vi "ObjDet_Read_Dataset_Single.vi"(6 "Dims(C,H,W)":T1={"C"=-1, "H"=-1, "W"=-1}, 7 "Unique labels":string[](array[string]), 8 "error in (no error)":errorcluster, 9 "Dataset Path (Images)":path=path "D:/DNN/Nuts_Bolts/Orig/1_Test/Images", 11 "Annotations Path":path=path "D:/DNN/Nuts_Bolts/Orig/1_Test/Annotations") -> (0 "error out":errorcluster, 2 "Anchors":dbl[][](array[numeric]), 3 "NN_DataSet(In3D_OutBBox)":T2={"Inputs Ref."=variant(refnum<data-value> refnum), "Dataset_Size"=0, "Dims_In"={"C"=0, "H"=0, "W"=0}, "Outputs Refs"=refnum, "No of Classes "=0, "Labels"=[], "File Paths"=[]})   [LabVIEW 2020]
uses:
  <vilib>/Ngene/Deep Learning Toolkit/Toolkit/NN_Data/API/DataSet/DataSet_Types/NN_DataSet(In3D_OutBBox).ctl
  <vilib>/Ngene/Deep Learning Toolkit/Toolkit/NN_Data/API/NN_Dims(C,H,W).ctl
  <vilib>/Ngene/Deep Learning Toolkit/Toolkit/NN_Data/Controls/DataRef_Types/1D/NN_Data_ref(1D_BBox).ctl
  <vilib>/Ngene/Deep Learning Toolkit/Toolkit/NN_Data/API/Data/Detection_Types/NN_Image_Annotations.ctl
  <vilib>/Ngene/Deep Learning Toolkit/Toolkit/NN_Data/API/Data/Detection_Types/NN_BBox_Annotation.ctl
  <vilib>/Ngene/Deep Learning Toolkit/Toolkit/NN_Data/API/Data/Detection_Types/NN_BBox.ctl
  <vilib>/Analysis/baseanly.llb/Mean (DBL).vi
  <vilib>/Ngene/Deep Learning Toolkit/Toolkit/Deep_Learning_Toolkit_by_Ngene.lvlib
  <vilib>/Analysis/NI_AALBase.lvlib
panel:
  out "Img Paths with missing Annotation":path[](array[path])
  out "Annotations with missing Imgs":path[](array[path])
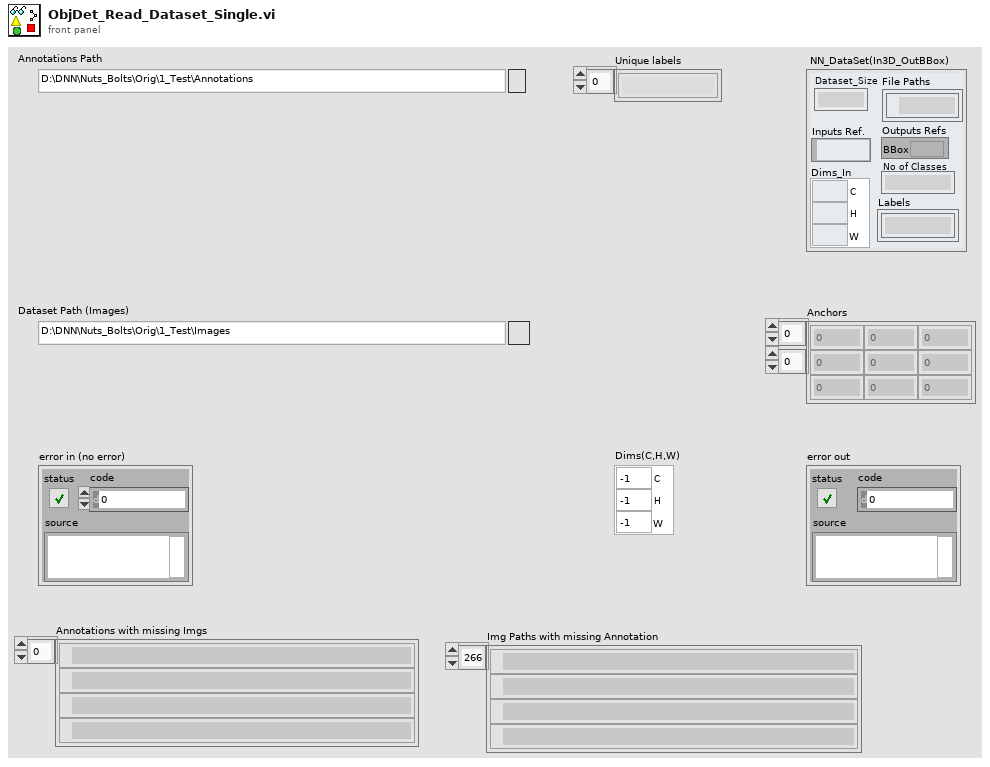
[diagram p1: front panel]
types:
  T1 = typedef "Deep_Learning_Toolkit_by_Ngene.lvlib/NN_Dims(C,H,W).ctl" = cluster{"C":i32, "H":i32, "W":i32}
  T2 = typedef "Deep_Learning_Toolkit_by_Ngene.lvlib/NN_DataSet(In3D_OutBBox).ctl" = cluster{"Inputs Ref.":variant, "Dataset_Size":i32, "Dims_In":T1, "Outputs Refs":T3, "No of Classes ":i32, "Labels":string[], "File Paths":path[]}
  T3 = typedef "Deep_Learning_Toolkit_by_Ngene.lvlib/NN_Data_ref(1D_BBox).ctl" = refnum<data-value>
  T4 = typedef "Deep_Learning_Toolkit_by_Ngene.lvlib/NN_Image_Annotations.ctl" = cluster{"Image Annotations":T5[]}
  T5 = typedef "Deep_Learning_Toolkit_by_Ngene.lvlib/NN_BBox_Annotation.ctl" = cluster{"Class":i32, "BBox":T6}
  T6 = typedef "Deep_Learning_Toolkit_by_Ngene.lvlib/NN_BBox.ctl" = cluster{"x":sgl, "y":sgl, "w":sgl, "h":sgl}
  T7 = typedef "Image Type" = u32
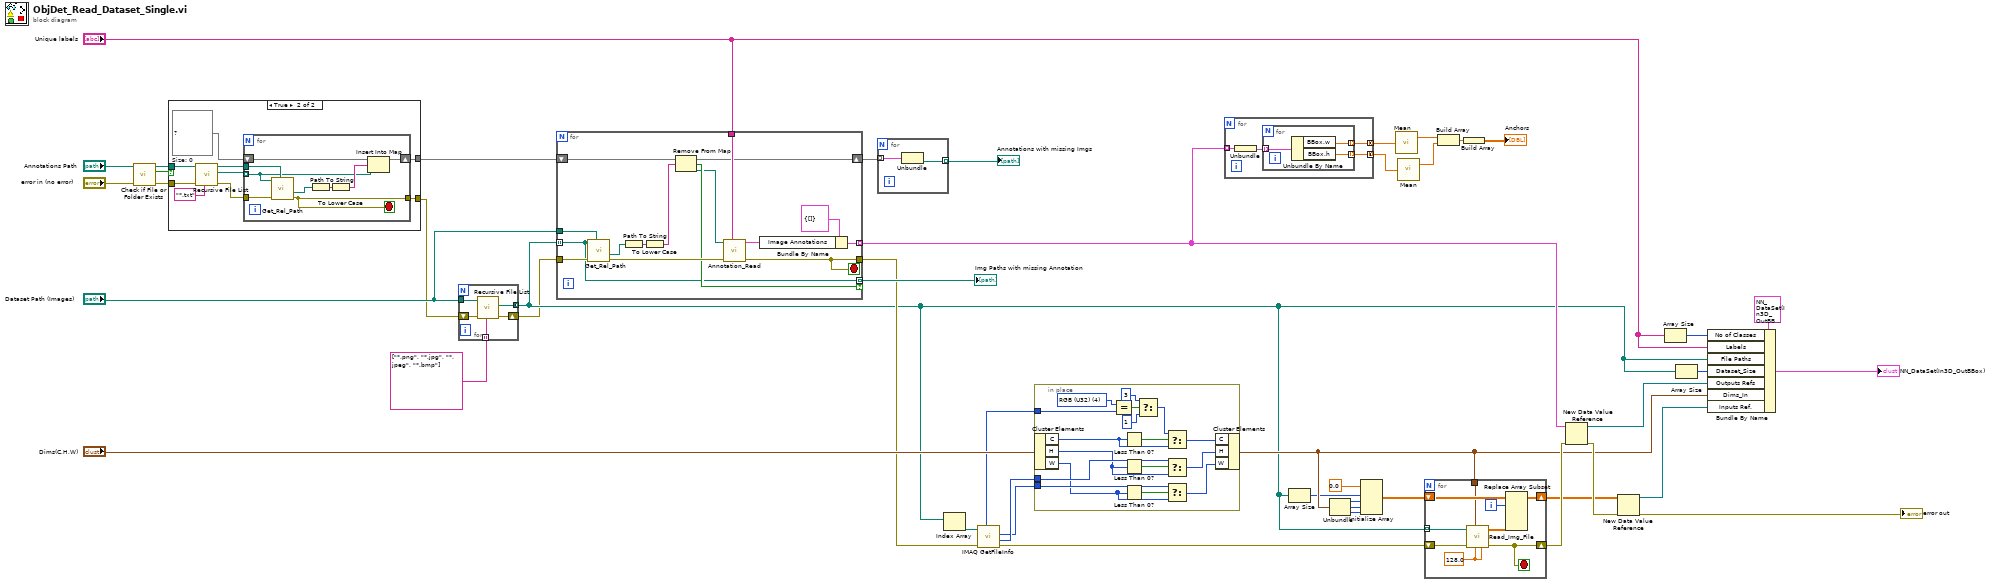
[diagram p0: block diagram]
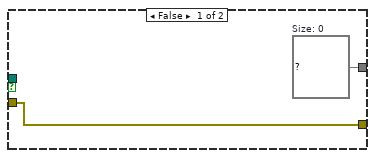
[diagram p2: hidden frame]
diagram:
  n1 = call <vilib>:"Check if File or Folder Exists.vi"("error in (no error)"="error in (no error)", "path"="Annotations Path") -> ("error out"=w3:errorcluster, "file or folder exists?"=w1:bool, "dup path"=w2:path)  [unwired: 7 in]
  n2 = case shown="True" w1 {
    tunnel: [w48 w53] -> w9
    tunnel: [w47 w51] -> w4
    tunnel: w3 -> [w47 w50]
    tunnel: w2 -> [_ w49]
    frame False {
      w48 = map{string, path} {}  # Size: 0
    }
    frame True {
      w54 = map{string, path} {}  # Size: 0
      n3 = call <vilib>:"Recursive File List.vi"("pattern"="*.txt", "error in (no error)"=w50, "Folder Path"=w49) -> ("error out"=w52:errorcluster, "All Files in Dir"=w56:path[], "dup Folder Path"=w55:path)  [unwired: 4 in, 2 out]
      n4 = for {
        tunnel: w56 -> [w60] mode=indexing
        shift-right: [w65] -> w53
        shift-left: w54 -> [w66]
        tunnel: w55 -> [w63]
        tunnel: w52 -> [w59]
        tunnel: [w58] -> w51
        stop <- w58 stop-if-true
        n5 = call "Get_Rel_Path.vi"("Parrent Folder"=w63, "error in (no error)"=w59, "Source File"=w60) -> ("error out"=w58:errorcluster, "Rel Path without extension"=w64:path)  [unwired: 5 in, 2 out]
        n6 = Path To String(path=w64) -> (string=w62:string)
        n7 = To Lower Case(string=w62) -> (all lower case string=w61:string)
        n8 = Insert Into Map(map in=w66, key=w61, value=w60) -> (map out=w65:map{string, path})  [unwired: 2 out]
      }
    }
  }
  n9 = for {
    tunnel: "Dataset Path (Images)" -> [w71]
    tunnel: string[] ["*.png", "*.jpg", "*.jpeg", "*.bmp"] ("pattern") -> [w70] mode=indexing
    tunnel: [w69] -> w6 mode=concatenating
    shift-right: [w67] -> w5
    shift-left: w4 -> [w68]
    n10 = call <vilib>:"Recursive File List.vi"("pattern"=w70, "error in (no error)"=w68, "Folder Path"=w71) -> ("error out"=w67:errorcluster, "All Files in Dir"=w69:path[])  [unwired: 4 in, 3 out]
  }
  n11 = for {
    tunnel: w6 -> [w73] mode=indexing
    tunnel: [w86] -> w10 mode=indexing
    tunnel: w5 -> [w83]
    tunnel: [w81] -> w11
    tunnel: [w73] -> w37 mode=indexing if=w76
    tunnel: "Unique labels" -> [w84]
    shift-right: [w75] -> w8
    shift-left: w9 -> [w80]
    tunnel: "Dataset Path (Images)" -> [w72]
    stop <- w81 stop-if-true
    n12 = call "Get_Rel_Path.vi"("Parrent Folder"=w72, "error in (no error)"=w83, "Source File"=w73) -> ("error out"=w82:errorcluster, "Rel Path without extension"=w78:path)  [unwired: 5 in, 2 out]
    n13 = Path To String(path=w78) -> (string=w79:string)
    n14 = To Lower Case(string=w79) -> (all lower case string=w77:string)
    n15 = Remove From Map(10:w77, 11:w80) -> (1:w74:path, 2:w76:bool, 3:w75:map{string, path})
    n16 = call "Annotation_Read.vi"("Unique labels"=w84, "error in (no error)"=w82, "Path"=w74) -> ("error out"=w81:errorcluster, "Annotations (CWH)"=w85:T5[])  [unwired: 6 in, 1 out]
    n17 = Bundle By Name(cluster=T4 {"Image Annotations"=[]} ("Image_Truths"), "Image Annotations"=w85) -> (w86:T4)
  }
  "Img Paths with missing Annotation" <- w37
  n18 = for {
    tunnel: w8 -> [w89] mode=indexing
    tunnel: [w88] -> w38 mode=indexing
    n19 = Unbundle(w89) -> (w88:path)  [unwired: 1 out]
  }
  "Annotations with missing Imgs" <- w38
  n20 = Index Array(array=w6) -> (element=w22:path)  [unwired: 1 in]
  n21 = call "IMAQ GetFileInfo"("error in (no error)"=w11, "File Path"=w22) -> ("error out"=w21:errorcluster, "Y Resolution"=w20:i32, "X Resolution"=w19:i32, "Image Type"=w18:T7)  [unwired: 3 in, 3 out]
  n22 = in-place {
    in-place-border: w20 -> [w106]
    in-place-border: w19 -> [w105]
    in-place-border: w18 -> [w95]
    w94 = T7 4 items=["Grayscale (U8)", "Grayscale (I16)", "Grayscale (SGL)", "Complex (CSG)", "RGB (U32)", "HSL (U32)", "RGB (U64)", "Grayscale (U16)"] ("x")
    n23 = in-place-cluster #1("Dims(C,H,W)") -> ("C"=w101:i32, "H"=w100:i32, "W"=w90:i32)
    n24 = Equal?(x=w94, y=w95) -> (x = y?=w96:bool)
    n25 = Less Than 0?(x=w101) -> (x < 0?=w102:bool)
    n26 = Less Than 0?(x=w100) -> (x < 0?=w104:bool)
    n27 = Less Than 0?(x=w90) -> (x < 0?=w103:bool)
    n28 = Select(t=3 ("H"), s=w96, f=1 ("H")) -> (s? t:f=w91:i32)
    n29 = Select(t=w91, s=w102, f=w101) -> (s? t:f=w99:i32)
    n30 = Select(t=w106, s=w104, f=w100) -> (s? t:f=w98:i32)
    n31 = Select(t=w105, s=w103, f=w90) -> (s? t:f=w97:i32)
    n32 = in-place-cluster #1("C"=w99, "H"=w98, "W"=w97) -> (w16:T1)
  }
  n33 = for {
    tunnel: w10 -> [w110] mode=indexing
    tunnel: [w108] -> w36 mode=concatenating
    tunnel: [w107] -> w35 mode=concatenating
    n34 = Unbundle(w110) -> ("Image Annotations"=w109:T5[])
    n35 = for {
      tunnel: w109 -> [w113] mode=indexing
      tunnel: [w112] -> w108 mode=indexing
      tunnel: [w111] -> w107 mode=indexing
      n36 = Unbundle By Name(w113) -> ("BBox.w"=w112:sgl, "BBox.h"=w111:sgl)
    }
  }
  n37 = Array Size(array=w6) -> (size(s)=w14:i32)
  n38 = Unbundle(w16) -> ("C"=w25:i32, "H"=w24:i32, "W"=w23:i32)
  n39 = Initialize Array(sgl 0.0 ("element"), w14, w25, w24, w23) -> (w27:sgl[][][][])
  n40 = call-poly <vilib>:"Mean.vi"("X"=w36) -> ("mean"=w34:dbl)  [unwired: 1 out]
  n41 = call-poly <vilib>:"Mean.vi"("X"=w35) -> ("mean"=w33:dbl)  [unwired: 1 out]
  n42 = for {
    tunnel: w6 -> [w115] mode=indexing
    shift-right: [w121] -> w26
    shift-left: w27 -> [w122]
    tunnel: w16 -> [w118]
    shift-right: [w117] -> w29
    shift-left: w21 -> [w119]
    i -> [w120]
    stop <- w117 stop-if-true
    w114 = sgl 128.0 ("Shift")
    n43 = call "Read_Img_File.vi"("Divider"=w114, "Shift"=w114, "Dims(C,H,W)"=w118, "error in (no error)"=w119, "Path"=w115) -> ("error out"=w117:errorcluster, "Image Data"=w116:sgl[][][])  [unwired: 3 in, 2 out]
    n44 = Replace Array Subset(array=w122, new element=w116, index (dim 0)=w120) -> (w121:sgl[][][][])  [unwired: 3 in]
  }
  n45 = Build Array(w34, w33) -> (w32:dbl[])
  n46 = Build Array(w32) -> (→"Anchors":dbl[][])
  n47 = New Data Value Reference(data value=w10, error in=w29) -> (data value reference=w17:refnum<data-value>, error out=w30:errorcluster)
  n48 = New Data Value Reference(data value=w26, error in=w30) -> (data value reference=w15:refnum<data-value>, error out=→"error out":errorcluster)
  n49 = Array Size(array="Unique labels") -> (size(s)=w12:i32)
  n50 = Array Size(array=w6) -> (size(s)=w13:i32)
  n51 = Bundle By Name(cluster=T2 {"Inputs Ref."=variant(refnum<data-value> refnum), "Dataset_Size"=0, "Dims_In"={"C"=0, "H"=0, "W"=0}, "Outputs Refs"=refnum, "No of Classes "=0, "Labels"=["large", "small"], "File Paths"=[]} ("Train DataSet"), "No of Classes"=w12, "Labels"="Unique labels", "File Paths"=w6, "Dataset_Size"=w13, "Outputs Refs"=w17, "Dims_In"=w16, "Inputs Ref."=w15) -> (→"NN_DataSet(In3D_OutBBox)":T2)
